vi "Configure Channel Delay.vi"(0 "DG645 in":refnum<class "DG645.lvclass">, 5 "Target Channel":T1, 7 "Reference Channel":T1, 9 "Delay (s)":dbl, 11 "error in (no error)":errorcluster) -> (4 "DG645 out":refnum<class "DG645.lvclass">, 15 "error out":errorcluster)   [LabVIEW 2018, in "DG645.lvlib" / "DG645.lvclass"]
uses:
  DG645.lvclass
  PPLs/Digital Delay Generator/Parent/Digital Delay Generator.lvlibp/Custom Controls/Channel.ctl
  DG645.lvclass/DG645.ctl
  <instrlib>/Stanford Research DG645/Stanford Research DG645.lvlib
  PPLs/Digital Delay Generator/Parent/Digital Delay Generator.lvlibp/Digital Delay Generator.lvclass
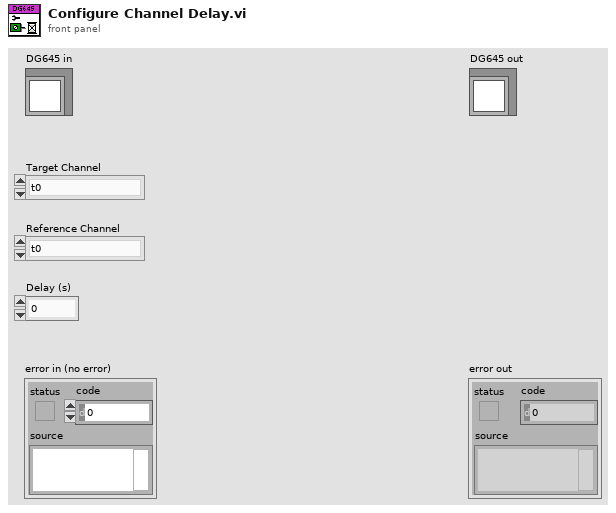
[diagram p1: front panel]
types:
  T1 = typedef "Digital Delay Generator.lvlibp/Digital Delay Generator.lvclass/Channel.ctl" = enum16{"t0", "A", "B", "C", "D", "E", "F", "G", "H"}
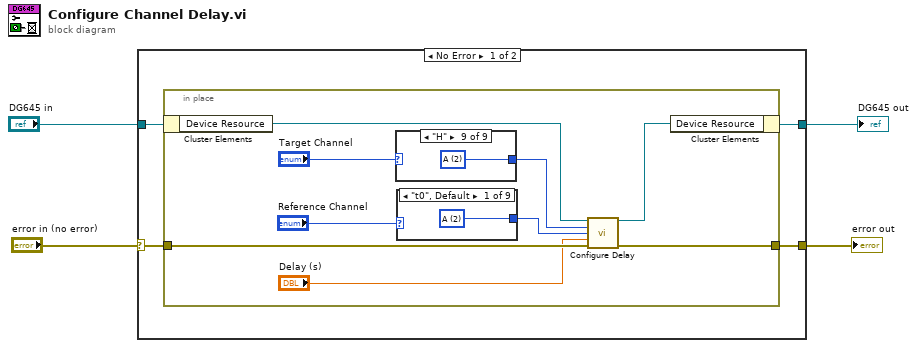
[diagram p0: block diagram]
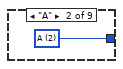
[diagram p2: hidden frame]
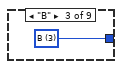
[diagram p3: hidden frame]
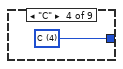
[diagram p4: hidden frame]
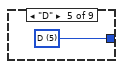
[diagram p5: hidden frame]
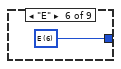
[diagram p6: hidden frame]
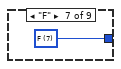
[diagram p7: hidden frame]
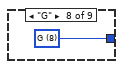
[diagram p8: hidden frame]
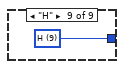
[diagram p9: hidden frame]
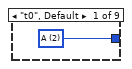
[diagram p10: hidden frame]
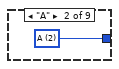
[diagram p11: hidden frame]
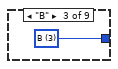
[diagram p12: hidden frame]
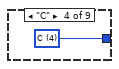
[diagram p13: hidden frame]
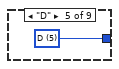
[diagram p14: hidden frame]
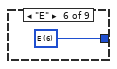
[diagram p15: hidden frame]
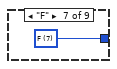
[diagram p16: hidden frame]
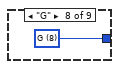
[diagram p17: hidden frame]
diagram:
  n1 = case shown="No Error" "error in (no error)" {
    selector: "error in (no error)" -> [w7 w36]
    tunnel: "DG645 in" -> [w8 w37]
    tunnel: [w6 w37] -> w2
    tunnel: [w5 w36] -> w1
    frame No Error {
      n2 = in-place {
        in-place-border: w7 -> [w17]
        in-place-border: [w13] -> w5
        n3 = in-place-cluster #1(w8) -> ("Device Resource"=w15:refnum<visa-resource-name>)
        n4 = case shown="\"H\"" "Target Channel" {
          tunnel: [w27 w28 w29 w30 w31 w32 w33 w34 w35] -> w9
          frame "t0", Default {
            w27 = u16 2 items=["A"=2, "B"=3, "C"=4, "D"=5, "E"=6, "F"=7, "G"=8, "H"=9] ("Channel to Modify (2:A)")
          }
          frame "A" {
            w28 = u16 2 items=["A"=2, "B"=3, "C"=4, "D"=5, "E"=6, "F"=7, "G"=8, "H"=9] ("Channel to Modify (2:A)")
          }
          frame "B" {
            w29 = u16 3 items=["A"=2, "B"=3, "C"=4, "D"=5, "E"=6, "F"=7, "G"=8, "H"=9] ("Channel to Modify (2:A)")
          }
          frame "C" {
            w30 = u16 4 items=["A"=2, "B"=3, "C"=4, "D"=5, "E"=6, "F"=7, "G"=8, "H"=9] ("Channel to Modify (2:A)")
          }
          frame "D" {
            w31 = u16 5 items=["A"=2, "B"=3, "C"=4, "D"=5, "E"=6, "F"=7, "G"=8, "H"=9] ("Channel to Modify (2:A)")
          }
          frame "E" {
            w32 = u16 6 items=["A"=2, "B"=3, "C"=4, "D"=5, "E"=6, "F"=7, "G"=8, "H"=9] ("Channel to Modify (2:A)")
          }
          frame "F" {
            w33 = u16 7 items=["A"=2, "B"=3, "C"=4, "D"=5, "E"=6, "F"=7, "G"=8, "H"=9] ("Channel to Modify (2:A)")
          }
          frame "G" {
            w34 = u16 8 items=["A"=2, "B"=3, "C"=4, "D"=5, "E"=6, "F"=7, "G"=8, "H"=9] ("Channel to Modify (2:A)")
          }
          frame "H" {
            w35 = u16 2 items=["A"=2, "B"=3, "C"=4, "D"=5, "E"=6, "F"=7, "G"=8, "H"=9] ("Channel to Modify (2:A)")
          }
        }
        n5 = case shown="\"t0\", Default" "Reference Channel" {
          tunnel: [w18 w19 w20 w21 w22 w23 w24 w25 w26] -> w10
          frame "t0", Default {
            w18 = u16 2 items=["T0"=0, "A"=2, "B"=3, "C"=4, "D"=5, "E"=6, "F"=7, "G"=8, "H"=9] ("Reference Channel (0:T0)")
          }
          frame "A" {
            w19 = u16 2 items=["T0"=0, "A"=2, "B"=3, "C"=4, "D"=5, "E"=6, "F"=7, "G"=8, "H"=9] ("Reference Channel (0:T0)")
          }
          frame "B" {
            w20 = u16 3 items=["T0"=0, "A"=2, "B"=3, "C"=4, "D"=5, "E"=6, "F"=7, "G"=8, "H"=9] ("Reference Channel (0:T0)")
          }
          frame "C" {
            w21 = u16 4 items=["T0"=0, "A"=2, "B"=3, "C"=4, "D"=5, "E"=6, "F"=7, "G"=8, "H"=9] ("Reference Channel (0:T0)")
          }
          frame "D" {
            w22 = u16 5 items=["T0"=0, "A"=2, "B"=3, "C"=4, "D"=5, "E"=6, "F"=7, "G"=8, "H"=9] ("Reference Channel (0:T0)")
          }
          frame "E" {
            w23 = u16 6 items=["T0"=0, "A"=2, "B"=3, "C"=4, "D"=5, "E"=6, "F"=7, "G"=8, "H"=9] ("Reference Channel (0:T0)")
          }
          frame "F" {
            w24 = u16 7 items=["T0"=0, "A"=2, "B"=3, "C"=4, "D"=5, "E"=6, "F"=7, "G"=8, "H"=9] ("Reference Channel (0:T0)")
          }
          frame "G" {
            w25 = u16 8 items=["T0"=0, "A"=2, "B"=3, "C"=4, "D"=5, "E"=6, "F"=7, "G"=8, "H"=9] ("Reference Channel (0:T0)")
          }
          frame "H" {
            w26 = u16 9 items=["T0"=0, "A"=2, "B"=3, "C"=4, "D"=5, "E"=6, "F"=7, "G"=8, "H"=9] ("Reference Channel (0:T0)")
          }
        }
        n6 = call <instrlib>:"Configure Delay.vi"("VISA resource name"=w15, "Channel to Modify (2:A)"=w9, "Reference Channel (0:T0)"=w10, "Delay Time (0 s)"="Delay (s)", "error in (no error)"=w17) -> ("VISA resource name out"=w14:refnum<visa-resource-name>, "error out"=w13:errorcluster)  [unwired: 9 in]
        n7 = in-place-cluster #1("Device Resource"=w14) -> (w6:refnum<class "DG645.lvclass">)
      }
    }
    frame Error {
    }
  }
  "error out" <- w1
  "DG645 out" <- w2
